vi "Abstract MVA Application Template.vi"   [LabVIEW 2018, in "MVA Framework.lvlib"]
uses:
  MVA Framework.lvlib
  modules/mva-core/Source/IModel/IModel/IModel.lvclass
  modules/mva-viewable/Source/IViewable/IViewable/IViewable.lvclass
  modules/mva-viewable/Source/IViewModel/IViewModel/IViewModel.lvclass
  C:/Program Files (x86)/National Instruments/LabVIEW 2018/vi.lib/ActorFramework/Actor/Actor.lvclass
  modules/mva-core/Source/MonitoredMediator/MonitoredMediator/MonitoredMediator.lvclass
  <vilib>/ActorFramework/Message Enqueuer/Message Priority.ctl
  modules/mva-viewable/Source/IViewable/IViewable/View Position Enum.ctl
  Source/BusMonitor/ListboxBusMonitor/ListboxBusMonitor/ListboxBusMonitor.lvclass/ListboxBusMonitor.ctl
  modules/mva-core/Source/MonitoredMediator/MonitoredMediator/MonitoredMediator.lvclass/MonitoredMediator.ctl
  modules/composed-event-logger/Source/Composed Log/LoggerReference/LoggerReference.lvclass/LoggerReference.ctl
  modules/mva-core/Source/IObserver/IObserver/IObserver.lvclass/IObserver.ctl
  modules/mva-core/Source/IMediator/IMediator/IMediator.lvclass/IMediator.ctl
  modules/mva-viewable/Source/IViewModel/IViewModel/IViewModel.lvclass/IViewModel.ctl
  modules/mva-viewable/Source/IViewManager/IViewManager Messages/Launch Nested Views Msg/Launch Nested Views Msg.lvclass/Launch Nested Views Msg.ctl
  modules/mva-viewable/Source/IViewManager/IViewManager/IViewManager.lvclass/IViewManager.ctl
  modules/mva-viewable/Source/IViewable/IViewable Messages/Open Front Panel Msg/Open Front Panel Msg.lvclass/Open Front Panel Msg.ctl
  <vilib>/ActorFramework/Message Enqueuer/Message Enqueuer.lvclass/Message Enqueuer.ctl
  8aeb1c73-ee09-4c42-9ba4-2ac02e328119.vi
  5c4f144a-bf04-4631-b5b9-56dc2cdea438.vi
  modules/mva-core/Source/MonitoredMediator/MonitoredMediator/Private Write BusMonitors.vi
  5c4f144a-bf04-4631-b5b9-56dc2cdea438.vi/4b58e03c-be92-4cd2-9125-f78d078cfd67.vi
  modules/mva-core/Source/IObserver/IObserver/Configure Observer Logging.vi
  modules/mva-viewable/Source/IViewModel/IViewModel/Write Startup Model-View Configuration.vi
  modules/mva-core/Source/IMediator/IMediator/Configure Mediator.vi
  <vilib>/ActorFramework/Message Enqueuer/Enqueue.vi
  modules/composed-event-logger/Source/Composed Log/LoggerReference/Return Aggregate Queues.vi
  modules/composed-event-logger/Source/Composed Log/LoggerReference/Add Aggregate Log.vi
  5c4f144a-bf04-4631-b5b9-56dc2cdea438.vi/4b58e03c-be92-4cd2-9125-f78d078cfd67.vi/467b9aba-ab44-4297-978f-72bf0771973b.vi
  modules/mva-viewable/Source/IViewManager/IViewManager Messages/Launch Nested Views Msg/Pack Launch Nested Views Msg.vi
  modules/mva-viewable/Source/IViewManager/IViewManager/Write Startup Launch Nested Views Msg.vi
  modules/composed-event-logger/Source/Composed Log/LoggerReference/Send Add Sink.vi
  modules/composed-event-logger/Source/Text File Sink/Text File Sink.lvclass
  modules/mva-viewable/Source/IViewable/IViewable Messages/Open Front Panel Msg/Open Front Panel Msg.lvclass
  C:/Program Files (x86)/National Instruments/LabVIEW 2018/vi.lib/ActorFramework/Message/Message.lvclass
  modules/composed-event-logger/Source/Composed Log/Application Logger/Launch Worker Loop.vi
  modules/composed-event-logger/Source/Composed Log/LoggerReference/Initialize Logger Instance.vi
  <vilib>/ActorFramework/Message Priority Queue/Priority Enqueue.vi
  Source/BusMonitor/ListboxBusMonitor/ListboxBusMonitor/ListboxBusMonitor.lvclass
  modules/mva-viewable/Source/IViewable/IApplicationStyle/IApplicationStyle.lvclass
  modules/composed-event-logger/Source/Composed Log/LoggerReference/LoggerReference.lvclass
  modules/composed-event-logger/Source/Composed Log/IErrorFormat/IErrorFormat.lvclass
  modules/composed-event-logger/Source/Composed Log/Log Sink/Log Sink.lvclass
  modules/mva-viewable/Source/IViewManager/IViewManager Messages/Launch Nested Views Msg/Launch Nested Views Msg.lvclass
  <vilib>/ActorFramework/Actor/Actor.lvclass
  <vilib>/ActorFramework/Message Enqueuer/Message Enqueuer.lvclass
panel:
  # "This example launches a simple abstract MVA application.\nReplace IModel with your Root Model or dependency-injected Model hierarchy.\nReplace IViewable with your Viewable or nested hierarchy of Viewables and ViewManagers\nReplace IViewModel with your concrete ViewModel that requests Model activity driven by user inputs\nMediator is already concrete--only replace it if you write your own Mediator"
types:
  T1 = typedef "MVA Framework.lvlib/IViewable.lvlib/IViewable.lvclass/View Position Enum.ctl" = enum16{"Centered", "Maximized", "Minimized", "Custom", "Unchanged"}
  T2 = typedef "Actor Framework.lvlib/Message Enqueuer.lvclass/Message Priority.ctl" = enum16{"Low", "Normal", "High"}
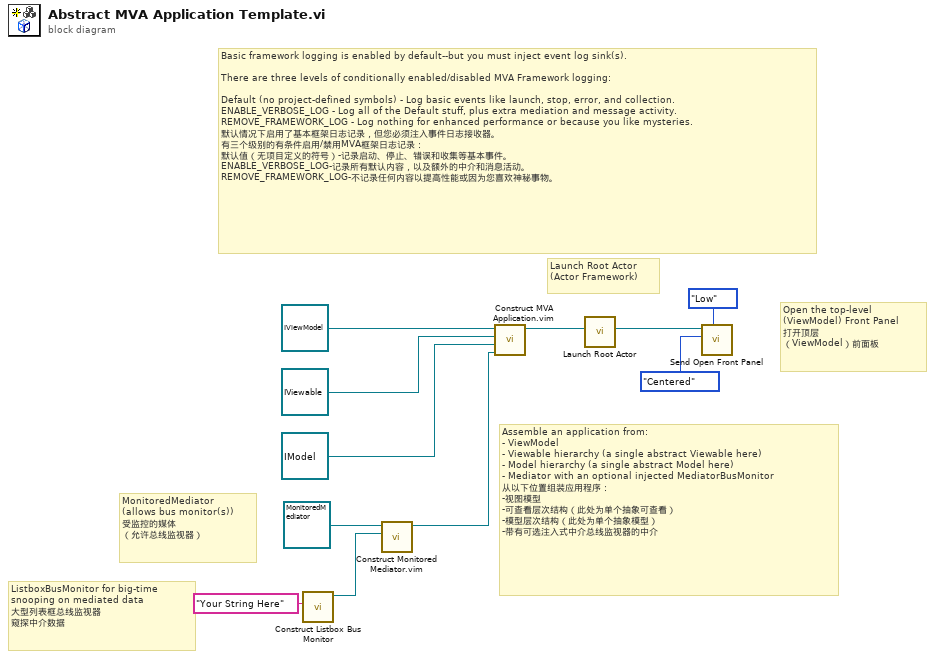
[diagram p0: block diagram]
diagram:
  # "ListboxBusMonitor for big-time\nsnooping on mediated data\n大型列表框总线监视器\n窥探中介数据"
  # "MonitoredMediator\n(allows bus monitor(s))\n受监控的媒体\n（允许总线监视器）"
  # "Basic framework logging is enabled by default--but you must inject event log sink(s).\n\nThere are three levels of conditionally enabled/disabled MVA Framework logging:\n\nDefault (no project-defined symbols) - Log basic events like launch, stop, error, and collection.\nENABLE_VERBOSE_LOG - Log all of the Default stuff, plus extra mediation and message activity.\nREMOVE_FRAMEWORK_LOG - Log nothing for enhanced performance or because you like mysteries.\n默认情况下启用了基本框架日志记录，但您必须注入事件日志接收器。\n有三个级别的有条件启用/禁用MVA框架日志记录：\n默认值（无项目定义的符号）-记录启动、停止、错误和收集等基本事件。\nENABLE_VERBOSE_LOG-记录所有默认内容，以及额外的中介和消息活动。\nREMOVE_FRAMEWORK_LOG-不记录任何内容以提高性能或因为您喜欢神秘事物。"
  # "Open the top-level\n(ViewModel) Front Panel\n打开顶层\n（ViewModel）前面板"
  # "Launch Root Actor\n(Actor Framework)"
  # "Assemble an application from:\n- ViewModel\n- Viewable hierarchy (a single abstract Viewable here)\n- Model hierarchy (a single abstract Model here)\n- Mediator with an optional injected MediatorBusMonitor\n从以下位置组装应用程序：\n-视图模型\n-可查看层次结构（此处为单个抽象可查看）\n-模型层次结构（此处为单个抽象模型）\n-带有可选注入式中介总线监视器的中介"
  n1 = call "Construct Listbox Bus Monitor.vi"("Show Panel Boolean Name"="Your String Here") -> ("ListboxBusMonitor out"=w4:refnum<class "ListboxBusMonitor.lvclass">)  [unwired: 10 in]
  n2 = call "Construct Monitored Mediator.vim"("Startup Bus Monitor(s)"=w4, "MonitoredMediator in"=refnum<class "MonitoredMediator.lvclass"> refnum ("MonitoredMediator.lvlib:MonitoredMediator.lvclass")) -> ("MonitoredMediator out"=w1:refnum<class "MonitoredMediator.lvclass">)  [unwired: 9 in]
  n3 = call "Construct MVA Application.vim"("Mediator Type"=w1, "Model Type"=refnum<class "IModel.lvclass"> refnum ("IModel.lvlib:IModel.lvclass"), "Startup View Configuration"=refnum<class "IViewable.lvclass"> refnum ("IViewable.lvlib:IViewable.lvclass"), "IViewModel In"=refnum<class "IViewModel.lvclass"> refnum ("IViewModel.lvlib:IViewModel.lvclass")) -> ("IViewModel Out"=w8:refnum<class "IViewModel.lvclass">)  [unwired: 7 in]
  n4 = call <vilib>:"Launch Root Actor.vi"("Actor"=w8) -> ("Actor's Enqueuer"=w2:refnum<class "Message Enqueuer.lvclass">)  [unwired: 9 in, 1 out]
  n5 = call "Send Open Front Panel.vi"("Message Priority (Normal)"=Message_Priority."Low", "Position"=View_Position_Enum."Centered", "Message Enqueuer"=w2) -> ()  [unwired: 7 in, 2 out]
